vi "Test_Burst_Commandlist.vi"() -> ()   [LabVIEW 2013, in "VI-Test.lvlib"]
uses:
  classes/Tests/Burst/Burst.lvclass
  lib/VI-Test.lvlib
panel:
  in  "Boolean":bool=TRUE
  out "parameters":string[][](table)
  out "error out":errorcluster
  out "Commandlist":string
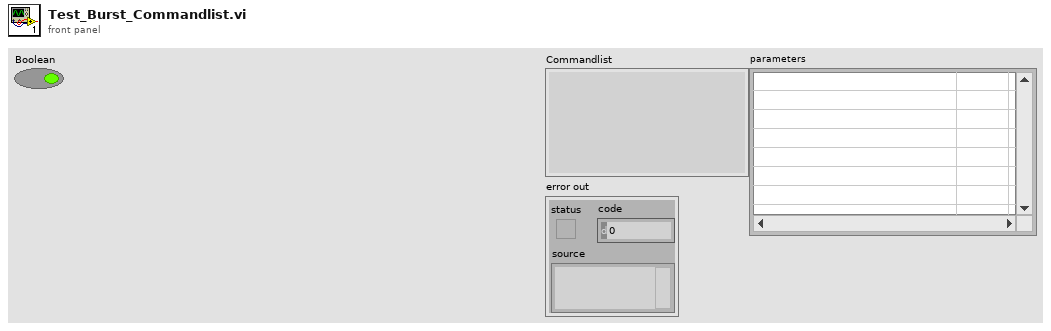
[diagram p1: front panel]
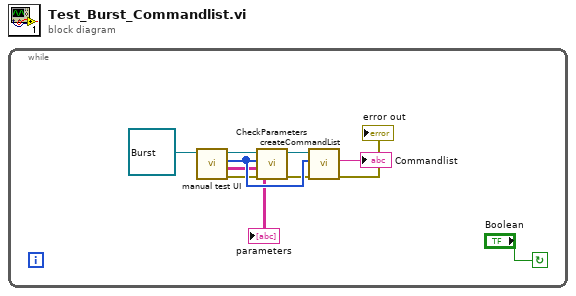
[diagram p0: block diagram]
diagram:
  n1 = while {
    stop <- "Boolean" continue-if-true
    n2 = call-dynamic "manual test UI.vi"("Burst Eingang"=refnum<class "Burst.lvclass"> refnum) -> ("error out"=w7:errorcluster, "parameters"=→"parameters":string[][], "Parameters"=w9:u32[], "Burst Ausgang"=w10:refnum<class "Burst.lvclass">)  [unwired: 6 in, 1 out]
    n3 = call-dynamic "CheckParameters.vi"("error in (no error)"=w7, "Parameters"=w9, "Burst in"=w10) -> ("error out"=w8:errorcluster, "Burst out"=w5:refnum<class "Burst.lvclass">)  [unwired: 7 in]
    n4 = call-dynamic "createCommandList.vi"("error in (no error)"=w8, "Parameters"=w9, "Burst in"=w5) -> ("error out"=→"error out":errorcluster, "Commandlist"=→"Commandlist":string)  [unwired: 6 in, 1 out]
  }
